vi "AnyBuilderBuildToBuffer.vi"(8 "error in (no error)":errorcluster, 10 "Message Type":string, 11 "Builder Ref":T1) -> (0 "error out":errorcluster, 3 "Buffer":u8[](array[numeric]))   [LabVIEW 2019, in "Template Server.lvlib" / "gprc-lvsupport.lvlib"]
uses:
  gprc-lvsupport.lvlib
  typeDefs/grpcId.ctl
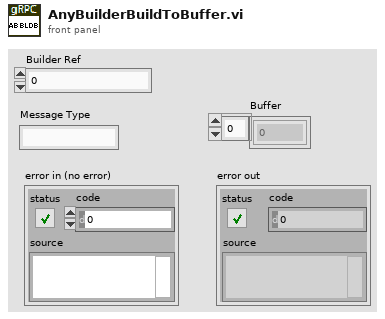
[diagram p1: front panel]
types:
  T1 = typedef "Template Server.lvlib/gprc-lvsupport.lvlib/grpcId.ctl" = u64
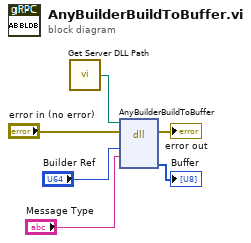
[diagram p0: block diagram]
diagram:
  n1 = call "Get Server DLL Path.vi"() -> ("Server dll path"=w5:path)
  n2 = dll-call lib="?" fn="AnyBuilderBuildToBuffer"(path in=w5, error in="error in (no error)", "builderId"="Builder Ref", "messageType"="Message Type") -> (error out=→"error out":errorcluster, "anyId"=→"Buffer":u8[])  [unwired: 5 in, 1 out]
